vi "sub_10lu_TabloBoya.vi"(2 "Table in":refnum<vi>, 3 "Tablo Degerleri":dbl[][](array[numeric])) -> (0 "Test Result":bool, 1 "RESULTS":string[](array[string]))   [LabVIEW 2014]
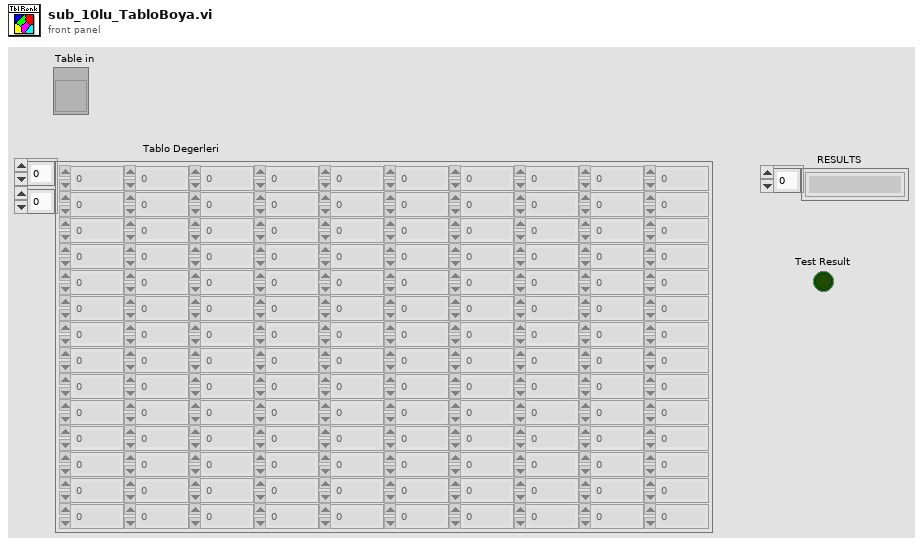
[diagram p1: front panel]
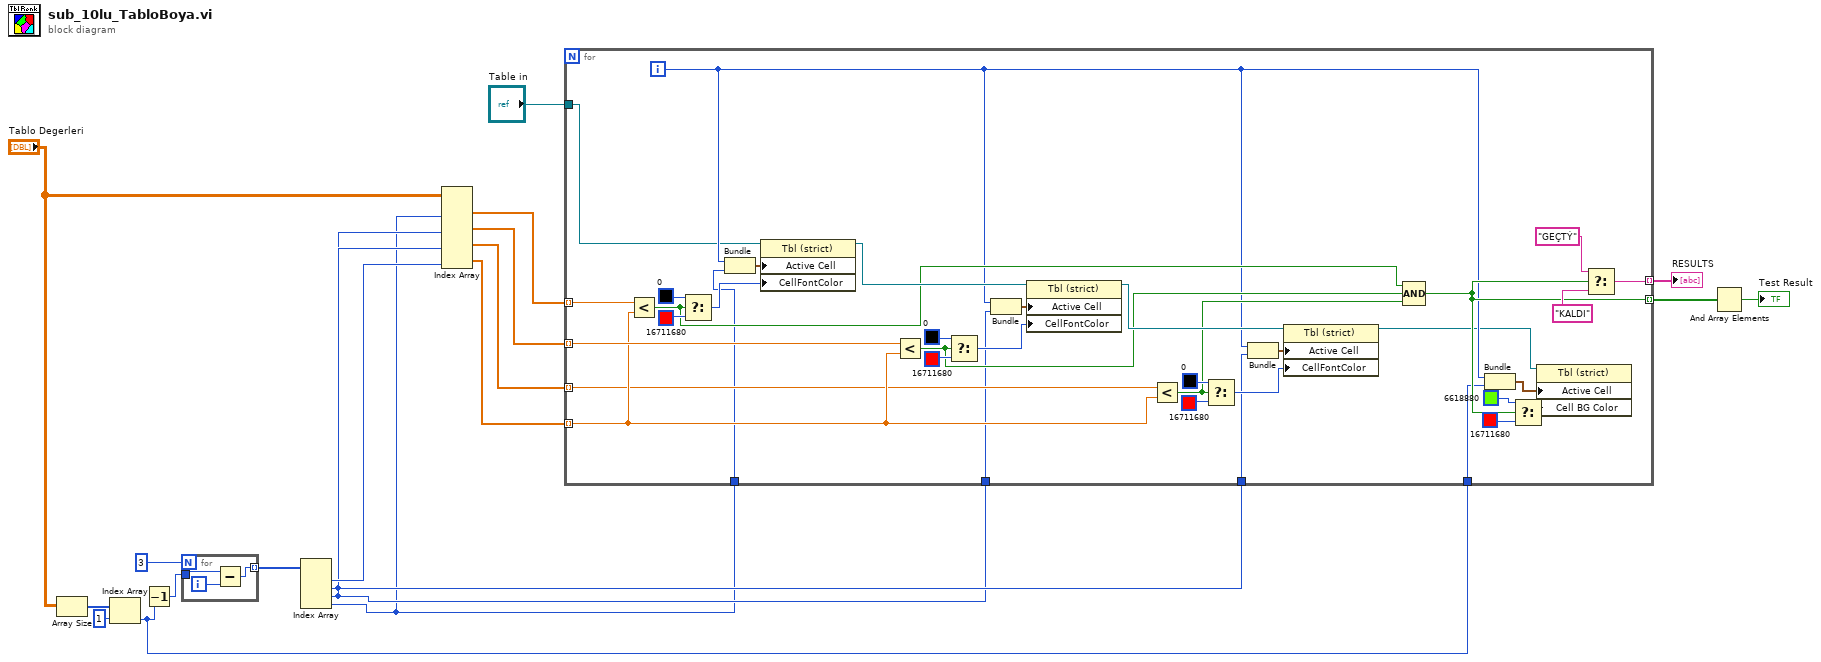
[diagram p0: block diagram]
diagram:
  n1 = Array Size(array="Tablo Degerleri") -> (size(s)=w10:i32[])
  n2 = Index Array(array=w10, index=1) -> (element=w4:i32)
  n3 = Decrement(x=w4) -> (x-1=w5:i32)
  n4 = for {
    N: 3 -> [_]
    tunnel: [w20] -> w8 mode=indexing
    tunnel: w5 -> [w21]
    i -> [w22]
    n5 = Subtract(x=w21, y=w22) -> (x-y=w20:i32)
  }
  n6 = Index Array(array=w8) -> (element #1=w6:i32, element #2=w3:i32, element #3=w2:i32, element #4=w1:i32)  [unwired: 4 in]
  n7 = Index Array(array="Tablo Degerleri", index (col) #1=w1, index (col) #2=w2, index (col) #3=w3, index (col) #4=w6) -> (element #1=w18:dbl[], element #2=w17:dbl[], element #3=w16:dbl[], element #4=w15:dbl[])  [unwired: 4 in]
  n8 = for {
    tunnel: "Table in" -> [w23]
    tunnel: w18 -> [w54] mode=indexing
    tunnel: w17 -> [w48] mode=indexing
    tunnel: w16 -> [w41] mode=indexing
    tunnel: w15 -> [w42] mode=indexing
    tunnel: [w35] -> w14 mode=indexing
    tunnel: [w34] -> w13 mode=indexing
    tunnel: w4 -> [w27]
    tunnel: w3 -> [w26]
    tunnel: w2 -> [w25]
    tunnel: w1 -> [w24]
    i -> [w30]
    n9 = Less?(x=w54, y=w42) -> (x < y?=w38:bool)
    n10 = Select(t=u32 0, s=w38, f=u32 16711680) -> (s? t:f=w56:u32)
    n11 = Bundle(w30, w24) -> (w55:cluster{i32, i32})  [unwired: 1 in]
    n12 = property on="Property Node" class="Tbl (strict)"(reference=w23, "Active Cell"=w55, "CellFontColor"=w56) -> (reference out=w49:refnum<vi>)  [unwired: 1 in, 1 out]
    n13 = Less?(x=w48, y=w42) -> (x < y?=w39:bool)
    n14 = Select(t=u32 0, s=w39, f=u32 16711680) -> (s? t:f=w51:u32)
    n15 = Bundle(w30, w25) -> (w50:cluster{i32, i32})  [unwired: 1 in]
    n16 = property on="Property Node" class="Tbl (strict)"(reference=w49, "Active Cell"=w50, "CellFontColor"=w51) -> (reference out=w43:refnum<vi>)  [unwired: 1 in, 1 out]
    n17 = Less?(x=w41, y=w42) -> (x < y?=w40:bool)
    n18 = Select(t=u32 0, s=w40, f=u32 16711680) -> (s? t:f=w45:u32)
    n19 = Bundle(w30, w26) -> (w44:cluster{i32, i32})  [unwired: 1 in]
    n20 = property on="Property Node" class="Tbl (strict)"(reference=w43, "Active Cell"=w44, "CellFontColor"=w45) -> (reference out=w28:refnum<vi>)  [unwired: 1 in, 1 out]
    n21 = Compound Arithmetic op=AND(w38, w39, w40) -> (w34:bool)
    n22 = Bundle(w30, w27) -> (w29:cluster{i32, i32})  [unwired: 1 in]
    n23 = Select(t=u32 6618880, s=w34, f=u32 16711680) -> (s? t:f=w31:u32)
    n24 = property on="Property Node" class="Tbl (strict)"(reference=w28, "Active Cell"=w29, "Cell BG Color"=w31) -> ()  [unwired: 1 in, 2 out]
    n25 = Select(t="GEÇTÝ", s=w34, f="KALDI") -> (s? t:f=w35:string)
  }
  "RESULTS" <- w14
  n26 = And Array Elements(Boolean array=w13) -> (logical AND=→"Test Result":bool)
